vi "Build message with Arguments.vi"() -> ()   [LabVIEW 2014]
uses:
  user.lib/_NEVSTOP/JKI State Machine++/_Polymophic/Build Register Status Message.vi
  user.lib/_NEVSTOP/JKI State Machine++/_Polymophic/Build Message with Arguments(Auto Check).vi
  user.lib/_NEVSTOP/JKI State Machine++/_Polymophic/Build No-Reply Asynchronous Message with Arguments.vi
  user.lib/_NEVSTOP/JKI State Machine++/_Polymophic/Build Asynchronous Message with Arguments.vi
  user.lib/_NEVSTOP/JKI State Machine++/_Polymophic/Build Synchronous Message with Arguments.vi
  user.lib/_NEVSTOP/JKI State Machine++/Utility/Trim Both Whitespace.vi
  user.lib/_NEVSTOP/JKI State Machine++/_Support/Message/Parse State with Arguments String.vi
  user.lib/_NEVSTOP/JKI State Machine++/JKI State Machine++.lvlib
panel:
  out "State with Arguments 18":string
  out "State with Arguments 17":string
  in  "Tab Control":T1(tab)
  out "State with Arguments":string
  out "State with Arguments 2":string
  out "State with Arguments 3":string
  out "State with Arguments 4":string
  out "State with Arguments 5":string
  out "State with Arguments 6":string
  out "State with Arguments 7":string
  out "State with Arguments 8":string
  out "State with Arguments 9":string
  out "State with Arguments 10":string
  out "State with Arguments 11":string
  out "State with Arguments 12":string
  out "State with Arguments 13":string
  out "State with Arguments 14":string
  out "State with Arguments 15":string
  out "State with Arguments 16":string
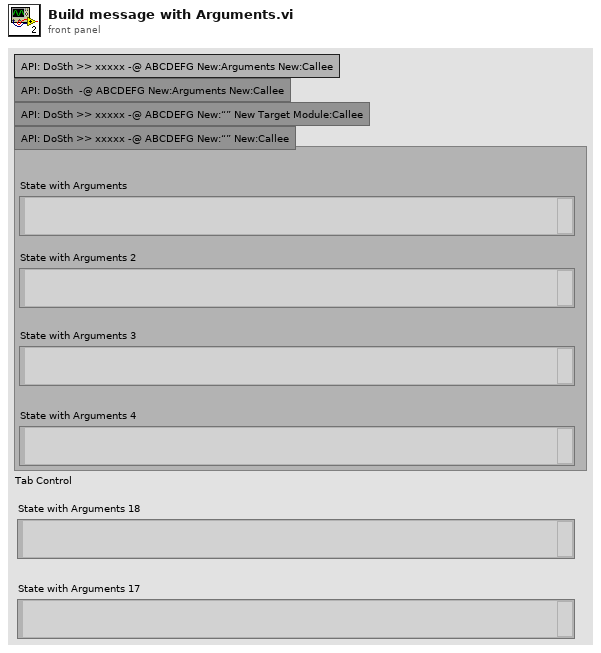
[diagram p1: front panel]
types:
  T1 = enum32{"API: DoSth >> xxxxx -@ ABCDEFG New:Arguments New:Callee", "API: DoSth  -@ ABCDEFG New:Arguments New:Callee", "API: DoSth >> xxxxx -@ ABCDEFG New:“” New Target Module:Callee", "API: DoSth >> xxxxx -@ ABCDEFG New:“” New:Callee"}
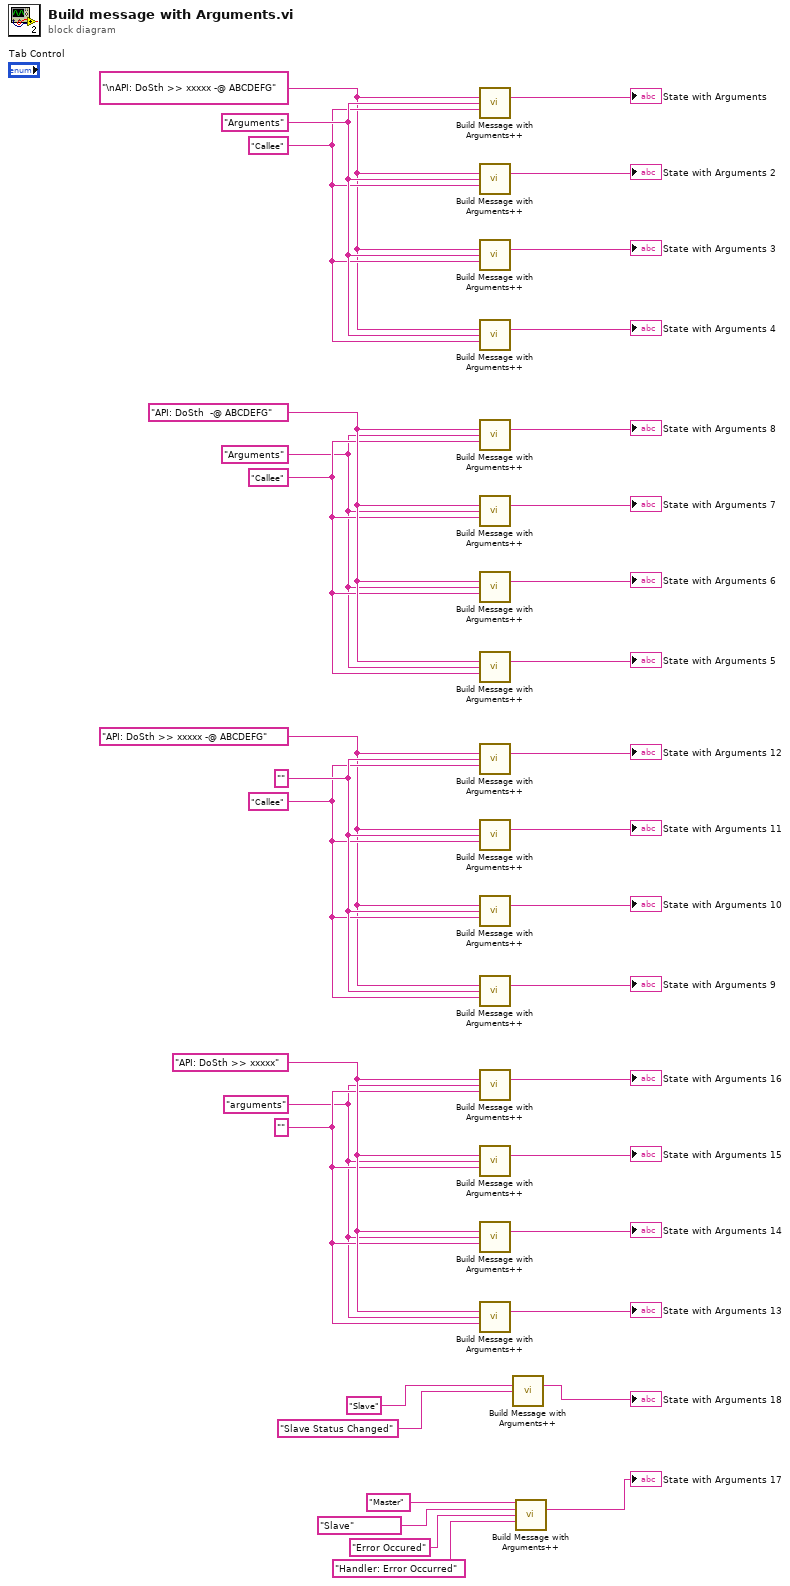
[diagram p0: block diagram]
diagram:
  w14 = "" ("State with Arguments")
  w13 = "arguments" ("State with Arguments")
  w15 = "API: DoSth >> xxxxx" ("State with Arguments")
  w17 = "Callee" ("State with Arguments")
  w18 = "" ("State with Arguments")
  w16 = "API: DoSth >> xxxxx -@ ABCDEFG" ("State with Arguments")
  w28 = "Callee" ("State with Arguments")
  w27 = "Arguments" ("State with Arguments")
  w29 = "API: DoSth  -@ ABCDEFG" ("State with Arguments")
  w31 = "Callee" ("State with Arguments")
  w32 = "Arguments" ("State with Arguments")
  w30 = "\nAPI: DoSth >> xxxxx -@ ABCDEFG" ("State with Arguments")
  n1 = call-poly "Build Message with Arguments++.vi"("State with Arguments"=w30, "Arguments (\"\")"=w32, "Target Module (\"\")"=w31) -> ("State with Arguments"=→"State with Arguments":string)  [unwired: 12 in]
  n2 = call-poly "Build Message with Arguments++.vi"("State with Arguments"=w30, "Arguments (\"\")"=w32, "Target Module (\"\")"=w31) -> ("State with Arguments"=→"State with Arguments 2":string)  [unwired: 12 in]
  n3 = call-poly "Build Message with Arguments++.vi"("State with Arguments"=w30, "Arguments (\"\")"=w32, "Target Module (\"\")"=w31) -> ("State with Arguments"=→"State with Arguments 3":string)  [unwired: 12 in]
  n4 = call-poly "Build Message with Arguments++.vi"("State with Arguments"=w30, "Arguments (\"\")"=w32, "Target Module (\"\")"=w31) -> ("State with Arguments"=→"State with Arguments 4":string)  [unwired: 12 in]
  n5 = call-poly "Build Message with Arguments++.vi"("State with Arguments"=w29, "Arguments (\"\")"=w27, "Target Module (\"\")"=w28) -> ("State with Arguments"=→"State with Arguments 8":string)  [unwired: 12 in]
  n6 = call-poly "Build Message with Arguments++.vi"("State with Arguments"=w29, "Arguments (\"\")"=w27, "Target Module (\"\")"=w28) -> ("State with Arguments"=→"State with Arguments 7":string)  [unwired: 12 in]
  n7 = call-poly "Build Message with Arguments++.vi"("State with Arguments"=w29, "Arguments (\"\")"=w27, "Target Module (\"\")"=w28) -> ("State with Arguments"=→"State with Arguments 6":string)  [unwired: 12 in]
  n8 = call-poly "Build Message with Arguments++.vi"("State with Arguments"=w29, "Arguments (\"\")"=w27, "Target Module (\"\")"=w28) -> ("State with Arguments"=→"State with Arguments 5":string)  [unwired: 12 in]
  n9 = call-poly "Build Message with Arguments++.vi"("State with Arguments"=w16, "Arguments (\"\")"=w18, "Target Module (\"\")"=w17) -> ("State with Arguments"=→"State with Arguments 12":string)  [unwired: 12 in]
  n10 = call-poly "Build Message with Arguments++.vi"("State with Arguments"=w16, "Arguments (\"\")"=w18, "Target Module (\"\")"=w17) -> ("State with Arguments"=→"State with Arguments 11":string)  [unwired: 12 in]
  n11 = call-poly "Build Message with Arguments++.vi"("State with Arguments"=w16, "Arguments (\"\")"=w18, "Target Module (\"\")"=w17) -> ("State with Arguments"=→"State with Arguments 10":string)  [unwired: 12 in]
  n12 = call-poly "Build Message with Arguments++.vi"("State with Arguments"=w16, "Arguments (\"\")"=w18, "Target Module (\"\")"=w17) -> ("State with Arguments"=→"State with Arguments 9":string)  [unwired: 12 in]
  n13 = call-poly "Build Message with Arguments++.vi"("State with Arguments"=w15, "Arguments (\"\")"=w13, "Target Module (\"\")"=w14) -> ("State with Arguments"=→"State with Arguments 16":string)  [unwired: 12 in]
  n14 = call-poly "Build Message with Arguments++.vi"("State with Arguments"=w15, "Arguments (\"\")"=w13, "Target Module (\"\")"=w14) -> ("State with Arguments"=→"State with Arguments 15":string)  [unwired: 12 in]
  n15 = call-poly "Build Message with Arguments++.vi"("State with Arguments"=w15, "Arguments (\"\")"=w13, "Target Module (\"\")"=w14) -> ("State with Arguments"=→"State with Arguments 14":string)  [unwired: 12 in]
  n16 = call-poly "Build Message with Arguments++.vi"("State with Arguments"=w15, "Arguments (\"\")"=w13, "Target Module (\"\")"=w14) -> ("State with Arguments"=→"State with Arguments 13":string)  [unwired: 12 in]
  n17 = call-poly "Build Message with Arguments++.vi"("Source JKISM Name (* as Default)"="Slave" ("Name(\"\" to use uuid)"), "Status"="Slave Status Changed" ("Message")) -> ("State with Arguments"=→"State with Arguments 18":string)  [unwired: 13 in]
  n18 = call-poly "Build Message with Arguments++.vi"("JKISM Name"="Master" ("Source JKISM Name"), "Source JKISM Name (* as Default)"="Slave" ("Name(\"\" to use uuid)"), "Status"="Error Occured" ("Message"), "Response Message (if \"\", same as Source Message)"="Handler: Error Occurred" ("Response Message (\"\" to use Message)")) -> ("State with Arguments"=→"State with Arguments 17":string)  [unwired: 11 in]
